vi "SCLN_IndexClient.vi"(1 "Server Name":string) -> (0 "Index":i32)   [LabVIEW 2015]
doc: "Find the index corresponding to\na client in the table of\nserver names. If the name doesn't exist, returns -1."
uses:
  SCLN_INT32_Select.ctl
  SCLN_RW_Select.ctl
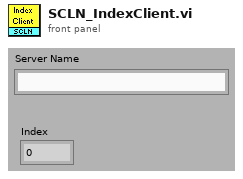
[diagram p1: front panel]
types:
  T1 = typedef "SCLN_RW_Select.ctl" = enum16{"Read", "Write"}
  T2 = typedef "SCLN_INT32_Select.ctl" = enum16{"Max_Servers", "Max_Clients", "Total_Servers", "Total_Clients"}
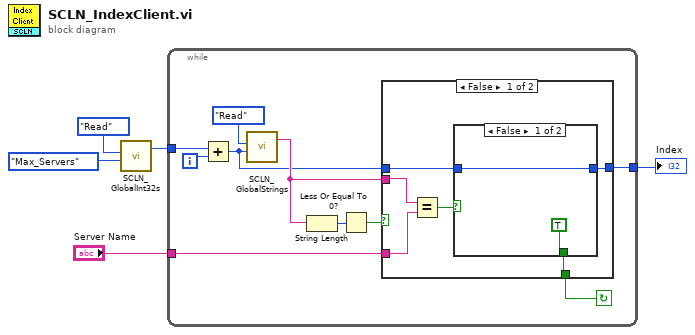
[diagram p0: block diagram]
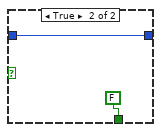
[diagram p2: hidden frame]
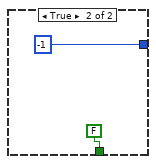
[diagram p3: hidden frame]
diagram:
  n1 = call "SCLN_GlobalInt32s.vi"("Element"=SCLN_INT32_Select."Max_Servers" ("GBL_INT32"), "Operation"=SCLN_RW_Select."Read" ("GBL_RW")) -> ("Read Value"=w1:i32)  [unwired: 2 in, 1 out]
  n2 = while {
    tunnel: [w12] -> w5
    tunnel: "Server Name" -> [w10]
    tunnel: w1 -> [w8]
    i -> [w7]
    stop <- w11 continue-if-true
    n3 = Add(x=w8, y=w7) -> (x+y=w6:i32)
    n4 = call "SCLN_GlobalStrings.vi"("Element"=w6, "Operation"=SCLN_RW_Select."Read" ("GBL_RW")) -> ("Read Value"=w9:string)  [unwired: 2 in, 1 out]
    n5 = String Length(string=w9) -> (length=w14:i32)
    n6 = Less Or Equal To 0?(x=w14) -> (x <= 0?=w13:bool)
    n7 = case shown="False" w13 {
      tunnel: [w17 -1] -> w12
      tunnel: [w16 FALSE] -> w11
      tunnel: w10 -> [w20 _]
      tunnel: w9 -> [w21 _]
      tunnel: w6 -> [w18 _]
      frame False {
        n8 = Equal?(x=w21, y=w20) -> (x = y?=w19:bool)
        n9 = case shown="False" w19 {
          tunnel: w18 -> [w22 w25]
          tunnel: [w22 w25] -> w17
          tunnel: [TRUE FALSE] -> w16
          frame False {
          }
          frame True {
          }
        }
      }
      frame True {
      }
    }
  }
  "Index" <- w5
